vi "ziGetEventVectorArray.vi"(7 "Error In":errorcluster, 9 "VectorWave In":T1, 10 "Handle In":T2 {"Handle" format="0x%08x"; "Conn" format="0x%08x"}) -> (0 "Error Out":errorcluster, 2 "VectorWave Out":T1, 3 "Handle Out":T2 {"Handle" format="0x%08x"; "Conn" format="0x%08x"})   [LabVIEW 2018, in "Zurich Instruments LabOne.lvlib"]
doc: "Decodes polled vector data from a Zurich Instruments device."
uses:
  Zurich Instruments LabOne.lvlib
  <instrlib>/Zurich Instruments LabOne/Private/ziLV64.framework
  ziTypeHandle.ctl
  ziTypeCoreVectorWave.ctl
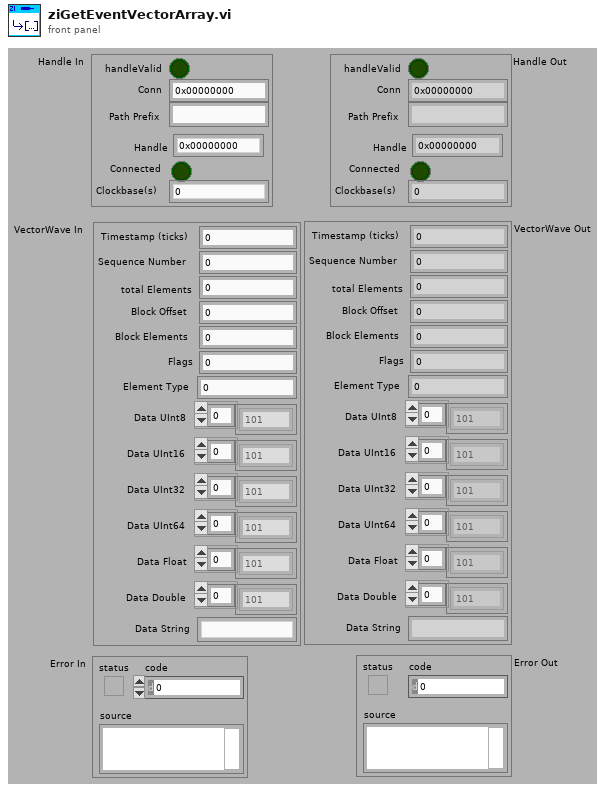
[diagram p1: front panel]
types:
  T1 = typedef "Zurich Instruments LabOne.lvlib/ziTypeCoreVectorWave.ctl" = cluster{"Timestamp (ticks)":u64, "Sequence Number":u32, "total Elements":u64, "Block Offset":u64, "Block Elements":u32, "Flags":u8, "Element Type":u8, "Data UInt8":u8[], "Data UInt16":u16[], "Data UInt32":u32[], "Data UInt64":u64[], "Data Float":sgl[], "Data Double":dbl[], "Data String":string}
  T2 = typedef "Zurich Instruments LabOne.lvlib/ziTypeHandle.ctl" = cluster{"handleValid":bool, "Conn":u64, "Path Prefix":string, "Handle":u64, "Connected":bool, "Clockbase(s)":dbl}
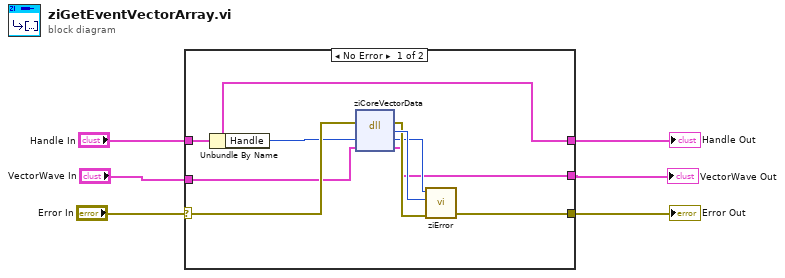
[diagram p0: block diagram]
diagram:
  n1 = case shown="No Error" "Error In" {
    selector: "Error In" -> [w14 w18]
    tunnel: "Handle In" -> [w10 w17]
    tunnel: [w10 w17] -> w5
    tunnel: [w15 w18] -> w4
    tunnel: [w8 w16] -> w2
    tunnel: "VectorWave In" -> [w7 w16]
    frame No Error {
      n2 = Unbundle By Name(w10) -> ("Handle"=w12:u64)
      n3 = dll-call lib="Applications/National Instruments/LabVIEW 2019 64-bit/instr.lib/Zurich Instruments LabOne/Private/ziLV*.*" fn="ziCoreVectorData" label="ziByteArrayToLV"(error in=w14, "ziEventBuffer"=w12, "byteArray"=w7) -> (error out=w11:errorcluster, "return type"=w13:u32, "ziEventBuffer"=w9:u64, "byteArray"=w8:T1)  [unwired: 2 in, 1 out]
      n4 = call "ziError.vi"("Conn"=w9, "ziErrorCode"=w13, "Error In"=w11) -> ("Error Out"=w15:errorcluster)  [unwired: 2 in, 1 out]
    }
    frame Error {
    }
  }
  "Handle Out" <- w5
  "Error Out" <- w4
  "VectorWave Out" <- w2
